vi "RobAndVision Calib.vi"() -> ()   [LabVIEW 2019]
uses:
  VisionSet/System/Ctrl/Photo.ctl
  VisionSet/System/Ctrl/Snap.ctl
  VisionSet/System/Ctrl/Grab.ctl
  <vilib>/vision/Image Controls.llb/IMAQ Image.ctl
  <vilib>/Utility/miscctls.llb/LVPositionTypeDef.ctl
  VisionSet/System/iVision/Controls/Parameter.ctl
  <vilib>/vision/Calibration.llb/Calibration Reference Points.ctl
  <vilib>/vision/Calibration.llb/Distortion Model.ctl
  <vilib>/vision/Calibration.llb/Distortion Model Types.ctl
  82d71f7b-eff0-4029-865a-31d7ef133adf.vi
  f2c65bda-5532-4734-abd4-11d5f743d3e2.vi
  7fbe03bc-4cd6-46c6-99fb-193606e1ede5.vi
  cee5a01b-f54d-48e6-866c-d4c8b1824800.vi
  57e8f32b-8e96-48c7-8808-a32c069fc57f.vi
  0d2cf41f-4f59-416b-aed8-33cf38611db5.vi
  d4251633-b06f-41b2-8266-4a47a039af55.vi
  f1238aa0-85ca-4192-9bd4-185fb6dc1a45.vi
  9afc25ec-97d4-45e3-b1ed-0db5aa0ecab6.vi
  3be21112-cc0e-4c3e-822b-1ce693b2e410.vi
  4e0eac2e-4d25-4abe-97ec-9d7757f58109.vi
  <vilib>/JDP Science/JSONtext/JSON text to Variant.vi
  VisionSet/System/iVision/Global/VisionGlb.vi
  <vilib>/JDP Science/JSONtext/Variant to JSON Text.vi
  LLB/Commonly VI.lvlib
  <vilib>/vision/NI_Vision_Development_Module.lvlib
panel:
  in  "Interpolation Type":u32(ring) items=["Zero Order", "Bi-Linear", "Quadratic", "Cubic Spline"]
  out "Calib Tem":T1
  in  "Seek Forward Button":bool
  in  "Seek Back Button":bool
  in  "Tab Control":enum32{"Page 1", "Page 2"}(tab)
  in  "Tab Control 3":enum32{"檢測圖", "校正圖"}(tab)
  out "Image":T1(plugin-control)
  out "Image 2":T1(plugin-control)
  in  "Btn_Save":bool
  in  "btn_Grab":T2
  in  "Btn_Snap":T3
  in  "Tab Control 2":enum32{"ToolData", "Vision&Robot"}(tab)
  in  "Tab Step":enum32{"Step1"}(tab)
  in  "ToolData":cluster{"X":dbl, "Y":dbl, "Angle":dbl}
  in  "RobotPos 2":cluster{"X":dbl, "Y":dbl, "Angle":dbl}
  in  "RobotPos 1":cluster{"X":dbl, "Y":dbl, "Angle":dbl}
  in  "UseCalib":bool caption="使用手臂坐標輸出"
  in  "ImgCalibration":bool caption="圖像校正"
  in  "PointName":u16(ring) caption="點位名稱" items=["1", "2", "3", "4", "5", "6", "7", "8", "9"]
  in  "btn_Search":bool
  in  "ProjectSet":u16(ring) caption="檢測設定專案"
  in  "Vision&Robot":T4(array[cluster])=[{"VisionPoint"={"X"=1142.846313, "Y"=534.709839}, "RobotPoint"={"X"=148.382, "Y"=73.831, "U"=0.0}}, {"VisionPoint"={"X"=2874.444336, "Y"=544.788269}, "RobotPoint"={"X"=351.458, "Y"=80.442, "U"=0.0}}, {"VisionPoint"={"X"=1132.611328, "Y"=1805.647461}, "RobotPoint"={"X"=152.021, "Y"=-80.98, "U"=0.0}}, {"VisionPoint"={"X"=2866.671875, "Y"=1821.208374}, "RobotPoint"={"X"=356.701, "Y"=-71.332, "U"=0.0}}, {"VisionPoint"={"X"=0.0, "Y"=0.0}, "RobotPoint"={"X"=0.0, "Y"=0.0, "U"=0.0}}, {"VisionPoint"={"X"=0.0, "Y"=0.0}, "RobotPoint"={"X"=0.0, "Y"=0.0, "U"=0.0}}, {"VisionPoint"={"X"=0.0, "Y"=0.0}, "RobotPoint"={"X"=0.0, "Y"=0.0, "U"=0.0}}]
  in  "相機":u16(ring) items=["cam0"]
  in  "Photo":T5
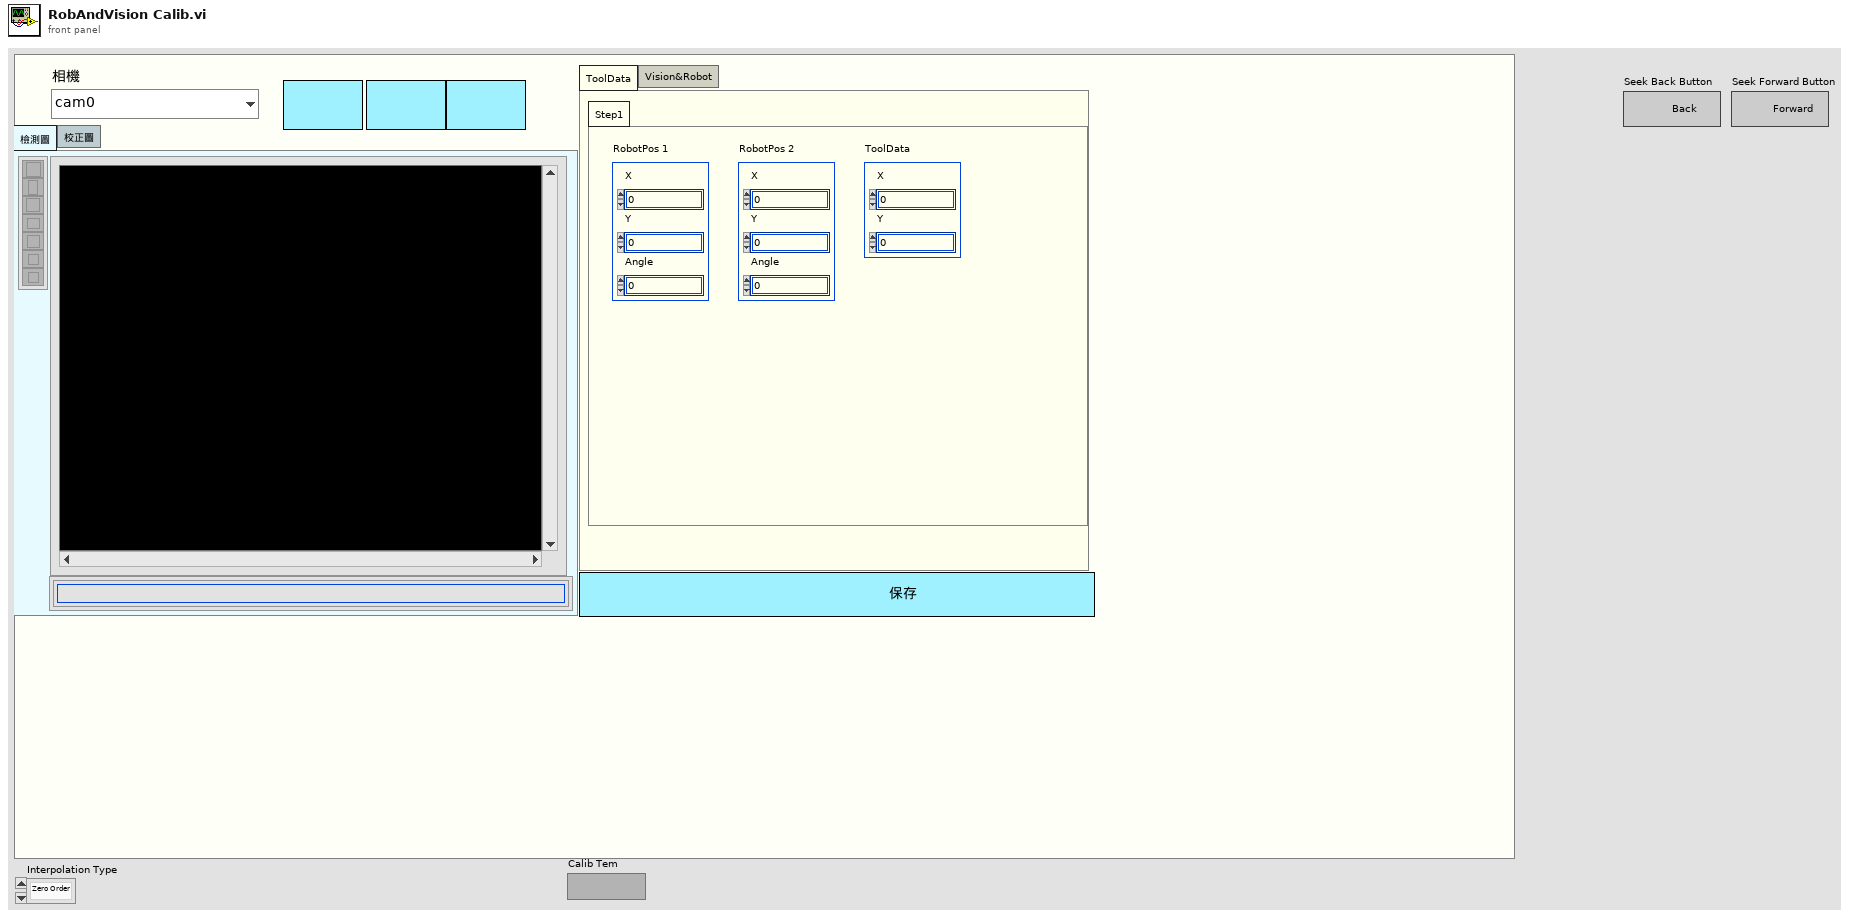
[diagram p1: front panel]
types:
  T1 = typedef "IMAQ Image.ctl" = refnum<image>
  T2 = typedef "Grab.ctl" = bool
  T3 = typedef "Snap.ctl" = bool
  T4 = cluster{"VisionPoint":cluster{"X":dbl, "Y":dbl}, "RobotPoint":cluster{"X":dbl, "Y":dbl, "U":dbl}}[]
  T5 = typedef "Photo.ctl" = bool
  T6 = typedef "LVPositionTypeDef.ctl" = cluster{"Left":i32, "Top":i32}
  T7 = enum16{"Initial", "Write", "Read", "Save", "Load", "WrteAll"}
  T8 = enum16{"initial", "write", "add", "delete", "Load", "Save", "Read", "ReadProjectName"}
  T9 = typedef "Parameter.ctl" = enum16{"Initialize", "Write", "Read", "WriteAll", "Save", "Load"}
  T10 = typedef "Distortion Model.ctl" = cluster{"Distortion Model":T11, "Polynomial Model Setup":cluster{"Radial Coefficient":u32, "Tangential Coefficients ":bool}}
  T11 = typedef "Distortion Model Types.ctl" = i32
  T12 = typedef "Image Unit" = enum32{"Undefined", "Angström", "Micrometer", "Millimeter", "Centimeter", "Meter", "Kilometer", "Microinch", "Inch", "Feet", "Nautical miles", "Standard miles", "Steps"}
  T13 = typedef "Calibration Reference Points.ctl" = cluster{"Pixel Coordinates":cluster{"X":dbl, "Y":dbl}[], "Real World Coordinates":cluster{"X":dbl, "Y":dbl}[], "Unit":T12, "Image Size":cluster{"X":u32, "Y":u32}}
  T14 = typedef "Image Type" = u32
  T15 = cluster{"0 Angle X Tool":dbl, "0 Angle Y Tool":dbl, dbl}
  T16 = typedef "ParameterData.ctl" = cluster{"Rotate Angle":dbl, "Rotate?":bool, "Calibration File Path":string, "Cal?":bool}
  T17 = cluster{"ProjectName":string, "Parameter":string[][]}
  T18 = cluster{"ROI":string, "Numbers":i32, "Data":string[][]}[]
  T19 = cluster{"VisionPoint":cluster{"X":dbl, "Y":dbl}, "RobotPoint":cluster{"X":dbl, "Y":dbl, "U":dbl}}
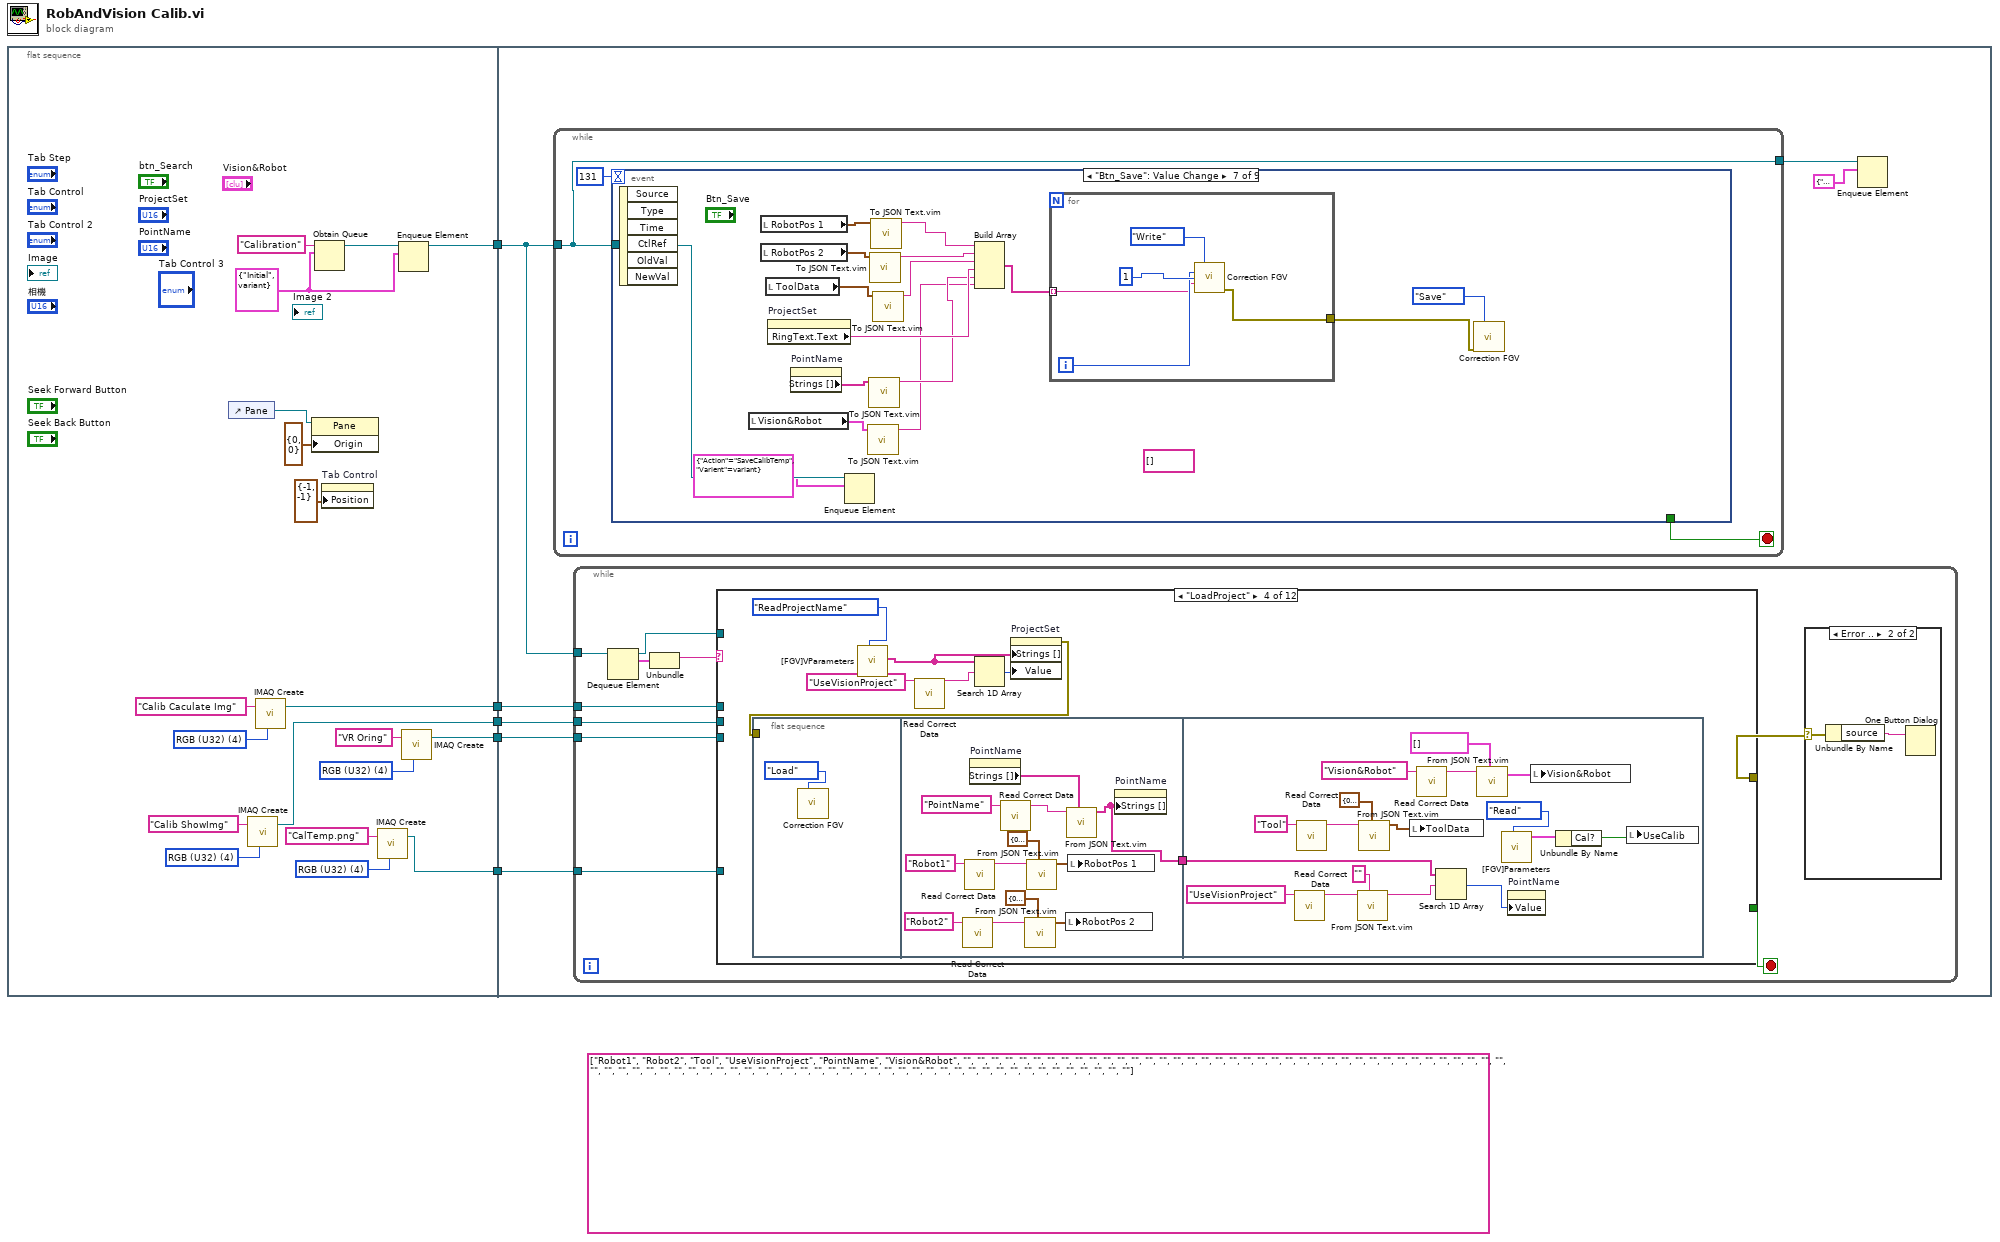
[diagram p0: block diagram]
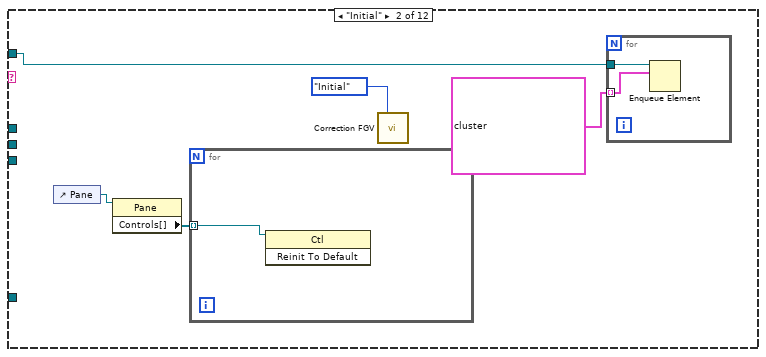
[diagram p4: hidden frame]
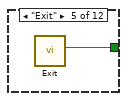
[diagram p6: hidden frame]
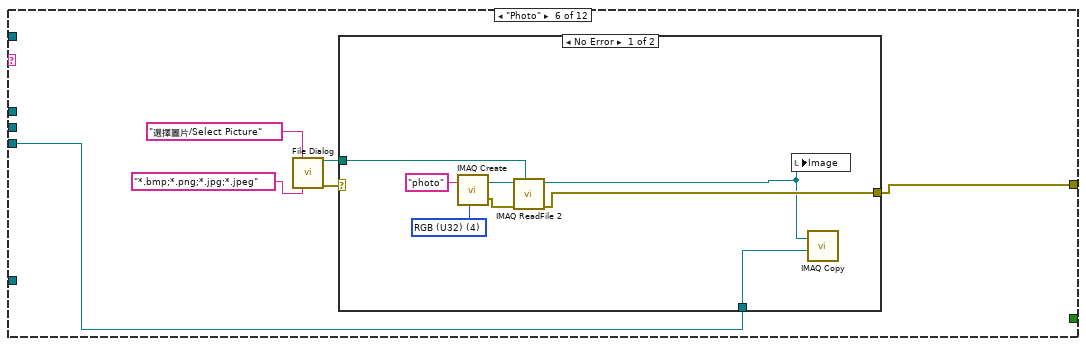
[diagram p7: hidden frame]
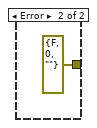
[diagram p8: hidden frame]
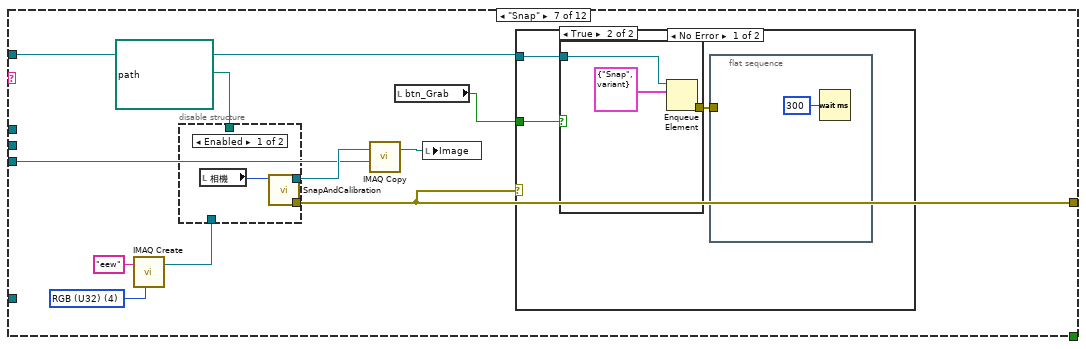
[diagram p9: hidden frame]
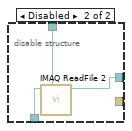
[diagram p10: hidden frame]
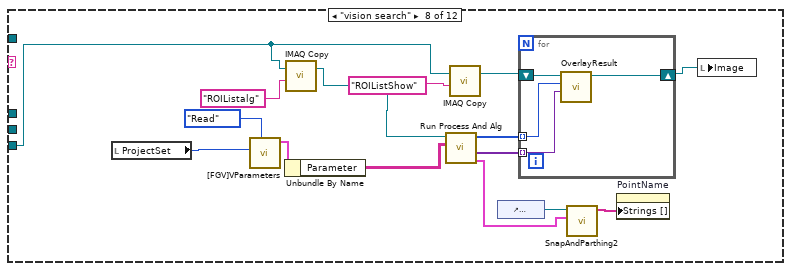
[diagram p13: hidden frame]
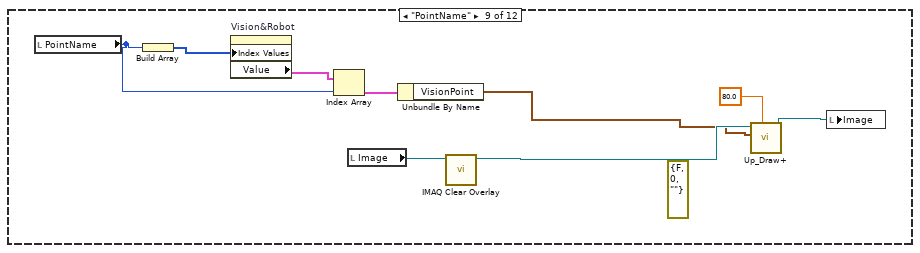
[diagram p14: hidden frame]
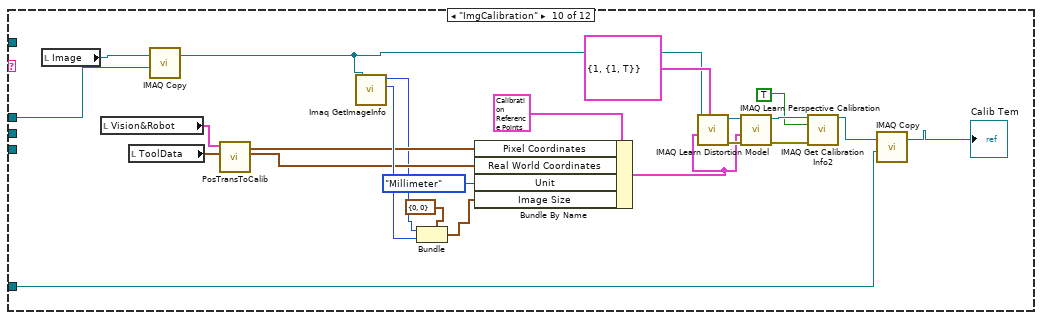
[diagram p15: hidden frame]
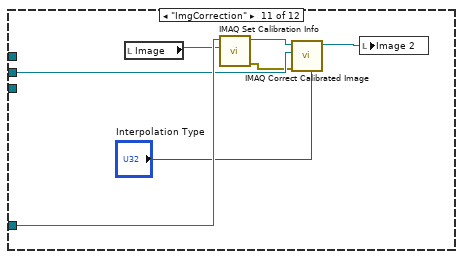
[diagram p16: hidden frame]
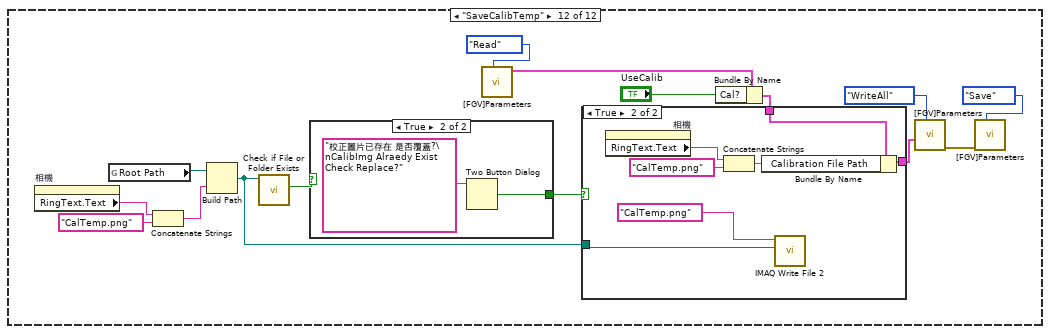
[diagram p17: hidden frame]
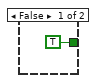
[diagram p19: hidden frame]
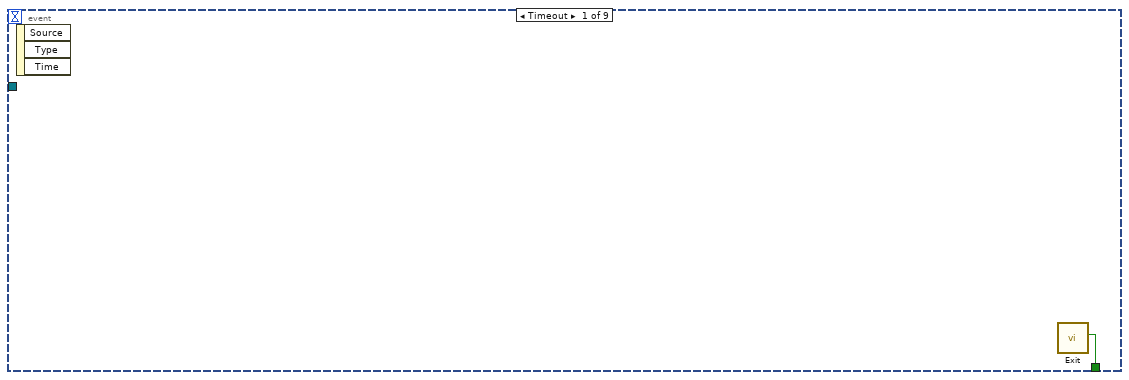
[diagram p20: hidden frame]
diagram:
  (unwired) string[][] [["Robot1", "Robot2", "Tool", "UseVisionProject", "PointName", "Vision&Robot", "", "", "", "", "", "", "", "", "", "", "", "", "", "", ""], ["", "", "", "", "", "", "", "", "", "", "", "", "", "", "", "", "", "", "", "", ""], ["", "", "", "", "", "", "", "", "", "", "", "", "", "", "", "", "", "", "", "", ""], ["", "", "", "", "", "", "", "", "", "", "", "", "", "", "", "", "", "", "", "", ""]] ("Item Names")
  n1 = flat-sequence {
    tunnel: [w22] -> w5
    tunnel: [w18] -> w4
    tunnel: [w12] -> w3
    tunnel: [w9] -> w2
    tunnel: [w6] -> w1
    tunnel: w5 -> [w30]
    tunnel: w4 -> [w28]
    tunnel: w3 -> [w27]
    tunnel: w2 -> [w26]
    tunnel: w1 -> [w25]
    frame #0 {
      w8 = T14 4 items=["Grayscale (U8)", "Grayscale (I16)", "Grayscale (SGL)", "Complex (CSG)", "RGB (U32)", "HSL (U32)", "RGB (U64)", "Grayscale (U16)"] ("Image Type")
      w10 = T14 4 items=["Grayscale (U8)", "Grayscale (I16)", "Grayscale (SGL)", "Complex (CSG)", "RGB (U32)", "HSL (U32)", "RGB (U64)", "Grayscale (U16)"] ("Image Type")
      w14 = T14 4 items=["Grayscale (U8)", "Grayscale (I16)", "Grayscale (SGL)", "Complex (CSG)", "RGB (U32)", "HSL (U32)", "RGB (U64)", "Grayscale (U16)"] ("Image Type")
      w19 = T14 4 items=["Grayscale (U8)", "Grayscale (I16)", "Grayscale (SGL)", "Complex (CSG)", "RGB (U32)", "HSL (U32)", "RGB (U64)", "Grayscale (U16)"] ("Image Type")
      w21 = cluster{"Action":string, "Varient":variant} {"Action"="Initial", "Varient"=variant} ("element")
      n2 = control-ref of="Pane"() -> (w17:refnum<vi>)
      n3 = call "IMAQ Create"("Image Name"="Calib ShowImg", "Image Type"=w8) -> ("New Image"=w6:T1)  [unwired: 3 in, 1 out]
      n4 = call "IMAQ Create"("Image Name"="Calib Caculate Img", "Image Type"=w10) -> ("New Image"=w9:T1)  [unwired: 3 in, 1 out]
      n5 = property class="Pane"(reference=w17, "Origin"=T6 {"Left"=0, "Top"=0} ("Position")) -> ()  [unwired: 1 in, 2 out]
      n6 = Obtain Queue(name (unnamed)="Calibration", element data type=w21) -> (queue out=w23:refnum<queue>)  [unwired: 3 in, 2 out]
      n7 = property on="Tab Control" class="TabCtl (strict)"("Position"=T6 {"Left"=-1, "Top"=-1}) -> ()  [unwired: 2 in, 2 out]
      n8 = call "IMAQ Create"("Image Name"="CalTemp.png", "Image Type"=w14) -> ("New Image"=w12:T1)  [unwired: 3 in, 1 out]
      n9 = Enqueue Element(queue=w23, element=w21) -> (queue out=w22:refnum<queue>)  [unwired: 2 in, 2 out]
      n10 = call "IMAQ Create"("Image Name"="VR Oring", "Image Type"=w19) -> ("New Image"=w18:T1)  [unwired: 3 in, 1 out]
    }
    frame #1 {
      n11 = while {
        tunnel: w30 -> [w212]
        tunnel: [w212] -> w31
        stop <- w214 stop-if-true
        n12 = event shown="[6] \"Btn_Save\": Value Change" {
          selector: _ -> [_ _ _ _ _ _ _ _ _]
          dyn-events: _ -> [_ _ _ _ _ _ _ _ _]
          timeout: 131 -> [_ _ _ _ _ _ _ _ _]
          tunnel: [w215 _ _ _ _ _ _ _ _] -> w214
          tunnel: w212 -> [_ w218 w220 w222 w224 w226 w230 _ w257]
          event Timeout {
            n13 = event-data() -> ()  [unwired: 1 in, 3 out]
            n14 = call "Exit.vi"() -> ("ExitOut"=w215:bool)  [unwired: 11 in]
          }
          event "btn_Search": Value Change {
            n15 = event-data() -> ()  [unwired: 1 in, 2 out]
            n16 = local write "btn_Grab"(T2 FALSE ("btn_Grab")) -> ()
            n17 = Enqueue Element(queue=w218, element=cluster{"Action":string, "Varient":variant} {"Action"="vision search", "Varient"=variant}) -> ()  [unwired: 2 in, 3 out]
          }
          event Value Change {
            n18 = event-data() -> ()  [unwired: 1 in, 6 out]
            n19 = Enqueue Element(queue=w220, element=cluster{"Action":string, "Varient":variant} {"Action"="Snap", "Varient"=variant}) -> ()  [unwired: 2 in, 3 out]
          }
          event Value Change {
            n20 = event-data() -> ()  [unwired: 1 in, 6 out]
            n21 = Enqueue Element(queue=w222, element=cluster{"Action":string, "Varient":variant} {"Action"="Snap", "Varient"=variant}) -> ()  [unwired: 2 in, 3 out]
          }
          event Value Change {
            n22 = event-data() -> ()  [unwired: 1 in, 1 out]
            n23 = Enqueue Element(queue=w224, element=cluster{"Action":string, "Varient":variant} {"Action"="Photo", "Varient"=variant}) -> ()  [unwired: 2 in, 3 out]
          }
          event "PointName": Value Change {
            n24 = event-data() -> ()  [unwired: 1 in, 3 out]
            n25 = Enqueue Element(queue=w226, element=cluster{"Action":string, "Varient":variant} {"Action"="PointName", "Varient"=variant}) -> ()  [unwired: 2 in, 3 out]
          }
          event "Btn_Save": Value Change {
            (unwired) string[] [] ("appended array")
            n26 = event-data() -> ()  [unwired: 1 in, 6 out]
            n27 = local read "Vision&Robot"() -> (w238:T4)
            n28 = local read "RobotPos 1"() -> (w242:cluster{"X":dbl, "Y":dbl, "Angle":dbl})
            n29 = local read "RobotPos 2"() -> (w241:cluster{"X":dbl, "Y":dbl, "Angle":dbl})
            n30 = local read "ToolData"() -> (w240:cluster{"X":dbl, "Y":dbl, "Angle":dbl})
            n31 = property on="ProjectSet" class="Ring (strict)"() -> ("RingText.Text"=w234:string)  [unwired: 2 in, 2 out]
            n32 = property on="PointName" class="Ring (strict)"() -> ("Strings []"=w239:string[])  [unwired: 2 in, 2 out]
            n33 = Enqueue Element(queue=w230, element=cluster{"Action":string, "Varient":variant} {"Action"="SaveCalibTemp", "Varient"=variant}) -> ()  [unwired: 2 in, 3 out]
            n34 = call "To JSON Text.vim"("Anything"=w238) -> ("<JSON>"=w232:string)  [unwired: 9 in, 1 out]
            n35 = call "To JSON Text.vim"("Anything"=w239) -> ("<JSON>"=w233:string)  [unwired: 9 in, 1 out]
            n36 = call "To JSON Text.vim"("Anything"=w241) -> ("<JSON>"=w236:string)  [unwired: 9 in, 1 out]
            n37 = call "To JSON Text.vim"("Anything"=w242) -> ("<JSON>"=w237:string)  [unwired: 9 in, 1 out]
            n38 = call "To JSON Text.vim"("Anything"=w240) -> ("<JSON>"=w235:string)  [unwired: 9 in, 1 out]
            n39 = Build Array(w237, w236, w235, w234, w233, w232) -> (w231:string[])
            n40 = for {
              tunnel: w231 -> [w244] mode=indexing
              tunnel: [w243] -> w227
              i -> [w245]
              n41 = call "Correction FGV.vi"("Action"=T7."Write", "X"=w245, "Y"=1, "DataIn"=w244) -> ("error out"=w243:errorcluster)  [unwired: 9 in, 2 out]
            }
            n42 = call "Correction FGV.vi"("Action"=T7."Save", "error in"=w227) -> ()  [unwired: 11 in, 3 out]
          }
          event "RobotPos 1", "RobotPos 2": Value Change {
            n43 = event-data() -> ()  [unwired: 1 in, 6 out]
            n44 = call "Robot Too Caculate.vi"("RobotPos 2"="RobotPos 2", "RobotPos 1"="RobotPos 1") -> ("0 Angle Y Tool"=w250:dbl, "0 Angle X Tool"=w251:dbl)  [unwired: 8 in]
            n45 = Bundle("0 Angle X Tool"=w251, "0 Angle Y Tool"=w250, 0.0) -> (w249:T15)  [unwired: 1 in]
            n46 = local write "ToolData"(w249) -> ()
          }
          event "ImgCalibration": Value Change {
            n47 = event-data() -> ()  [unwired: 1 in, 2 out]
            n48 = Enqueue Element(queue=w257, element=cluster{"Action":string, "Varient":variant} {"Action"="ImgCalibration", "Varient"=variant}) -> (queue out=w255:refnum<queue>)  [unwired: 2 in, 2 out]
            n49 = Enqueue Element(queue=w255, element=cluster{"Action":string, "Varient":variant} {"Action"="ImgCorrection", "Varient"=variant}) -> ()  [unwired: 2 in, 3 out]
          }
        }
      }
      n50 = while {
        tunnel: w30 -> [w41]
        tunnel: w28 -> [w37]
        tunnel: w27 -> [w34]
        tunnel: w26 -> [w33]
        tunnel: w25 -> [w32]
        stop <- w38 stop-if-true
        n51 = Dequeue Element(queue=w41) -> (queue out=w35:refnum<queue>, element=w40:cluster{"Action":string, "Varient":variant})  [unwired: 2 in, 2 out]
        n52 = Unbundle(w40) -> ("Action"=w39:string)  [unwired: 1 out]
        n53 = case shown="\"LoadProject\"" w39 {
          tunnel: [_ _ _ _ w89 _ _ _ _ _ _ _] -> w38
          tunnel: w37 -> [_ _ _ _ _ w90 w113 w136 _ _ _ _]
          tunnel: [_ _ _ _ _ w91 w111 _ _ _ _ _] -> w36
          tunnel: w35 -> [_ w46 _ _ _ _ w110 _ _ _ _ _]
          tunnel: w34 -> [_ _ _ _ _ _ _ _ _ w163 w185 _]
          tunnel: w33 -> [_ _ _ _ _ _ _ _ _ w160 _ _]
          tunnel: w32 -> [_ _ _ _ _ _ _ _ _ _ w181 _]
          frame "False", Default {
          }
          frame "Initial" {
            n54 = control-ref of="Pane"() -> (w48:refnum<vi>)
            n55 = property class="Pane"(reference=w48) -> ("Controls[]"=w47:refnum<vi>[])  [unwired: 1 in, 2 out]
            n56 = for {
              tunnel: w47 -> [w51] mode=indexing
              n57 = invoke class="Ctl" method="Reinit To Default"(reference=w51) -> ()  [unwired: 2 in, 3 out]
            }
            n58 = call "Correction FGV.vi"("Action"=T7."Initial") -> ()  [unwired: 12 in, 3 out]
            n59 = for {
              tunnel: w46 -> [w50]
              tunnel: cluster{"Action":string, "Varient":variant}[] [{"Action"="GetRoot", "Varient"=variant}, {"Action"="LoadProject", "Varient"=variant}] -> [w49] mode=indexing
              n60 = Enqueue Element(queue=w50, element=w49) -> ()  [unwired: 2 in, 3 out]
            }
          }
          frame "GetRoot" {
          }
          frame "LoadProject" {
            n61 = flat-sequence {
              tunnel: w53 -> [_]
              tunnel: [w60] -> w52
              tunnel: w52 -> [w74]
              frame #0 {
                n62 = call "Correction FGV.vi"("Action"=T7."Load") -> ()  [unwired: 12 in, 3 out]
              }
              frame #1 {
                n63 = call "Read Correct Data.vi"("DataName"="Robot2") -> ("DataOut"=w62:string)  [unwired: 10 in]
                n64 = call "Read Correct Data.vi"("DataName"="Robot1") -> ("DataOut"=w67:string)  [unwired: 10 in]
                n65 = property on="PointName" class="Ring (strict)"() -> ("Strings []"=w69:string[])  [unwired: 2 in, 2 out]
                n66 = call "Read Correct Data.vi"("DataName"="PointName") -> ("DataOut"=w70:string)  [unwired: 10 in]
                n67 = call "From JSON Text.vim"("Data Type and Default Value"=cluster{"X":dbl, "Y":dbl, "Angle":dbl} {"X"=0.0, "Y"=0.0, "Angle"=0.0} ("RobotPos 1"), "JSON"=w62) -> ("Data out"=w64:cluster{"X":dbl, "Y":dbl, "Angle":dbl})  [unwired: 8 in, 1 out]
                n68 = call "From JSON Text.vim"("Data Type and Default Value"=cluster{"X":dbl, "Y":dbl, "Angle":dbl} {"X"=0.0, "Y"=0.0, "Angle"=0.0} ("RobotPos 1"), "JSON"=w67) -> ("Data out"=w65:cluster{"X":dbl, "Y":dbl, "Angle":dbl})  [unwired: 8 in, 1 out]
                n69 = local write "RobotPos 2"(w64) -> ()
                n70 = call "From JSON Text.vim"("Data Type and Default Value"=w69, "JSON"=w70) -> ("Data out"=w60:string[])  [unwired: 8 in, 1 out]
                n71 = local write "RobotPos 1"(w65) -> ()
                n72 = property on="PointName" class="Ring (strict)"("Strings []"=w60) -> ()  [unwired: 2 in, 2 out]
              }
              frame #2 {
                n73 = call "Read Correct Data.vi"("DataName"="UseVisionProject") -> ("DataOut"=w77:string)  [unwired: 10 in]
                n74 = call "Read Correct Data.vi"("DataName"="Tool") -> ("DataOut"=w83:string)  [unwired: 10 in]
                n75 = call "From JSON Text.vim"("Data Type and Default Value"="" ("Ring Text.Text"), "JSON"=w77) -> ("Data out"=w73:string)  [unwired: 8 in, 1 out]
                n76 = call "From JSON Text.vim"("Data Type and Default Value"=cluster{"X":dbl, "Y":dbl, "Angle":dbl} {"X"=0.0, "Y"=0.0, "Angle"=0.0} ("RobotPos 1"), "JSON"=w83) -> ("Data out"=w81:cluster{"X":dbl, "Y":dbl, "Angle":dbl})  [unwired: 8 in, 1 out]
                n77 = local write "ToolData"(w81) -> ()
                n78 = call "Read Correct Data.vi"("DataName"="Vision&Robot") -> ("DataOut"=w87:string)  [unwired: 10 in]
                n79 = Search 1D Array(1D array=w74, element=w73) -> (index of element=w72:i32)  [unwired: 1 in]
                n80 = call "From JSON Text.vim"("Data Type and Default Value"=T4 [] ("Vision&Robot"), "JSON"=w87) -> ("Data out"=w88:T4)  [unwired: 8 in, 1 out]
                n81 = call "[FGV]Parameters.vi"("Parameter"=Parameter."Read") -> ("ParameterData Out"=w79:T16)  [unwired: 9 in, 1 out]
                n82 = property on="PointName" class="Ring (strict)"("Value"=w72) -> ()  [unwired: 2 in, 2 out]
                n83 = local write "Vision&Robot"(w88) -> ()
                n84 = Unbundle By Name(w79) -> ("Cal?"=w78:bool)
                n85 = local write "UseCalib"(w78) -> ()
              }
            }
            n86 = call "[FGV]VParameters.vi"("Enum"=T8."ReadProjectName") -> ("ProjectName"=w54:string[])  [unwired: 7 in, 3 out]
            n87 = call "Read Correct Data.vi"("DataName"="UseVisionProject") -> ("DataOut"=w57:string)  [unwired: 10 in]
            n88 = Search 1D Array(1D array=w54, element=w57) -> (index of element=w56:i32)  [unwired: 1 in]
            n89 = property on="ProjectSet" class="Ring (strict)"("Strings []"=w54, "Value"=w56) -> (error out=w53:errorcluster)  [unwired: 2 in, 1 out]
          }
          frame "Exit" {
            n90 = call "Exit.vi"() -> ("ExitOut"=w89:bool)  [unwired: 11 in]
          }
          frame "Photo" {
            n91 = call "File Dialog"("prompt"="選擇圖片/Select Picture", "pattern (all files)"="*.bmp;*.png;*.jpg;*.jpeg" ("pattern label")) -> ("selected path"=w95:path, "error out"=w94:errorcluster)  [unwired: 10 in, 2 out]
            n92 = case shown="No Error" w94 {
              tunnel: w95 -> [w100 _]
              tunnel: [w98 errorcluster {"status"=FALSE, "code"=0, "source"=""} ("error out")] -> w91
              tunnel: w90 -> [w97 _]
              frame No Error {
                w103 = T14 4 items=["Grayscale (U8)", "Grayscale (I16)", "Grayscale (SGL)", "Complex (CSG)", "RGB (U32)", "HSL (U32)", "RGB (U64)", "Grayscale (U16)"] ("Image Type")
                n93 = call "IMAQ Create"("Image Name"="photo", "Image Type"=w103) -> ("New Image"=w101:T1, "error out"=w99:errorcluster)  [unwired: 3 in]
                n94 = call "IMAQ ReadFile 2"("File Path"=w100, "error in (no error)"=w99, "Image"=w101) -> ("error out"=w98:errorcluster, "Image Out"=w96:T1)  [unwired: 4 in, 3 out]
                n95 = local write "Image"(w96) -> ()
                n96 = call "IMAQ Copy"("Image Dst"=w97, "Image Src"=w96) -> ()  [unwired: 4 in, 2 out]
              }
              frame Error {
              }
            }
          }
          frame "Snap" {
            w107 = T14 4 items=["Grayscale (U8)", "Grayscale (I16)", "Grayscale (SGL)", "Complex (CSG)", "RGB (U32)", "HSL (U32)", "RGB (U64)", "Grayscale (U16)"] ("Image Type")
            n97 = call "IMAQ Create"("Image Name"="eew", "Image Type"=w107) -> ("New Image"=w106:T1)  [unwired: 3 in, 1 out]
            n98 = disable-structure shown="Enabled" {
              disable-tunnel: [w116 w120] -> w114
              disable-tunnel: [w115 _] -> w111
              disable-tunnel: w106 -> [_ w119]
              disable-tunnel: path "C:/Users/USER/Desktop/PATTERN - 複製.png" ("File Path") -> [_ w118]
              frame Enabled {
                n99 = local read "相機"() -> (w117:u16)
                n100 = call "SnapAndCalibration.vi"("Value"=w117) -> ("error out"=w115:errorcluster, "Image Dst Out"=w116:T1)  [unwired: 9 in]
              }
              frame Disabled {
                n101 = call "IMAQ ReadFile 2"("File Path"=w118, "Image"=w119) -> ("Image Out"=w120:T1)  [unwired: 5 in, 4 out]
              }
            }
            n102 = call "IMAQ Copy"("Image Dst"=w113, "Image Src"=w114) -> ("Image Dst Out"=w112:T1)  [unwired: 4 in, 1 out]
            n103 = local read "btn_Grab"() -> (w109:T2)
            n104 = local write "Image"(w112) -> ()
            n105 = case shown="No Error" w111 {
              tunnel: w110 -> [w123 _]
              tunnel: w109 -> [w121 _]
              frame No Error {
                n106 = case shown="True" w121 {
                  tunnel: w123 -> [_ w125]
                  tunnel: [_ w124] -> w122
                  frame False {
                  }
                  frame True {
                    n107 = Enqueue Element(queue=w125, element=cluster{"Action":string, "Varient":variant} {"Action"="Snap", "Varient"=variant}) -> (error out=w124:errorcluster)  [unwired: 2 in, 2 out]
                  }
                }
                n108 = flat-sequence {
                  tunnel: w122 -> [_]
                  frame #0 {
                    n109 = Wait (ms)(milliseconds to wait=u32 300) -> ()  [unwired: 1 out]
                  }
                }
              }
              frame Error {
              }
            }
          }
          frame "vision search" {
            n110 = local read "ProjectSet"() -> (w134:u16)
            n111 = call "[FGV]VParameters.vi"("Enum"=T8."Read", "ProjectIndex"=w134) -> ("DataOut"=w133:T17)  [unwired: 6 in, 3 out]
            n112 = Unbundle By Name(w133) -> ("Parameter"=w132:string[][])
            n113 = call "IMAQ Copy"("Image Dst"="ROIListalg" ("Image Name"), "Image Src"=w136) -> ("Image Dst Out"=w138:T1)  [unwired: 4 in, 1 out]
            n114 = call "Run Process And Alg.vi"("ROIList"=w132, "Image"=w138) -> ("Result Arr"=w129:T18, "DetectOut"=w141:variant[], "AlgOut"=w140:i32[])  [unwired: 5 in, 2 out]
            n115 = call "IMAQ Copy"("Image Dst"="ROIListShow" ("Image Name"), "Image Src"=w136) -> ("Image Dst Out"=w142:T1)  [unwired: 4 in, 1 out]
            n116 = control-ref of="Vision&Robot"() -> (w130:refnum<vi>)
            n117 = for {
              tunnel: w141 -> [w145] mode=indexing
              shift-right: [w144] -> w131
              shift-left: w142 -> [w146]
              tunnel: w140 -> [w143] mode=indexing
              n118 = call "OverlayResult.vi"("DectectResult"=w145, "Algorithm"=w143, "Image"=w146) -> ("Image Out"=w144:T1)  [unwired: 8 in]
            }
            n119 = call "SnapAndParthing2.vi"("Result Arr"=w129, "Vision&Robot"=w130) -> ("Name"=w128:string[])  [unwired: 9 in]
            n120 = property on="PointName" class="Ring (strict)"("Strings []"=w128) -> ()  [unwired: 2 in, 2 out]
            n121 = local write "Image"(w131) -> ()
          }
          frame "PointName" {
            (unwired) errorcluster {"status"=FALSE, "code"=0, "source"=""} ("error out")
            n122 = local read "PointName"() -> (w153:u16)
            n123 = Build Array(w153) -> (w155:u16[])
            n124 = property on="Vision&Robot" class="Arr (strict)"("Index Values"=w155) -> ("Value"=w154:T4)  [unwired: 2 in, 2 out]
            n125 = Index Array(array=w154, index=w153) -> (element=w152:T19)
            n126 = local read "Image"() -> (w151:T1)
            n127 = Unbundle By Name(w152) -> ("VisionPoint"=w149:cluster{"X":dbl, "Y":dbl})
            n128 = call "IMAQ Clear Overlay"("Image"=w151) -> ("Image Out"=w150:T1)  [unwired: 9 in, 1 out]
            n129 = call "Up_Draw+.vi"("y"=80.0, "Center"=w149, "Image"=w150) -> ("Image Out"=w148:T1)  [unwired: 8 in]
            n130 = local write "Image"(w148) -> ()
          }
          frame "ImgCalibration" {
            n131 = local read "Image"() -> (w161:T1)
            n132 = local read "Vision&Robot"() -> (w156:T4)
            n133 = local read "ToolData"() -> (w157:cluster{"X":dbl, "Y":dbl, "Angle":dbl})
            n134 = call "IMAQ Copy"("Image Dst"=w160, "Image Src"=w161) -> ("Image Dst Out"=w159:T1)  [unwired: 4 in, 1 out]
            n135 = call "PosTransToCalib.vi"("ToolData"=w157, "Vision&Robot"=w156) -> ("Real"=w165:cluster{"X":dbl, "Y":dbl}[], "Vision"=w166:cluster{"X":dbl, "Y":dbl}[])  [unwired: 8 in]
            n136 = call "Imaq GetImageInfo"("Image"=w159) -> ("Y Resolution"=w168:i32, "X Resolution"=w158:i32)  [unwired: 3 in, 6 out]
            n137 = Bundle(cluster=cluster{"X":u32, "Y":u32} {"X"=0, "Y"=0} ("Image Size"), "X"=w158, "Y"=w168) -> (w169:cluster{"X":u32, "Y":u32})
            n138 = Bundle By Name(cluster=T13 {"Pixel Coordinates"=[{"X"=1144.0, "Y"=516.0}, {"X"=2876.7, "Y"=527.688}, {"X"=1131.38, "Y"=1786.7}, {"X"=2923.83, "Y"=1804.95}], "Real World Coordinates"=[{"X"=148.386, "Y"=76.831}, {"X"=351.958, "Y"=82.394}, {"X"=152.021, "Y"=-78.481}, {"X"=356.701, "Y"=-69.132}], "Unit"=enum."Millimeter", "Image Size"={"X"=3840, "Y"=2748}} ("Reference Points"), "Pixel Coordinates"=w166, "Real World Coordinates"=w165, "Unit"=Image_Unit."Millimeter", "Image Size"=w169) -> (w171:T13)
            n139 = call "IMAQ Learn Distortion Model"("Distortion Model Setup"=T10 {"Distortion Model"=1, "Polynomial Model Setup"={"Radial Coefficient"=1, "Tangential Coefficients "=TRUE}}, "Reference Points"=w171, "Calibration Template Image"=w159) -> ("error out"=w174:errorcluster, "Calibration Template Image Out"=w177:T1)  [unwired: 3 in, 4 out]
            n140 = call "IMAQ Learn Perspective Calibration"("error in (no error)"=w174, "Reference Points"=w171, "Calibration Template Image"=w177) -> ("error out"=w173:errorcluster, "Calibration Template Image Out"=w176:T1)  [unwired: 1 in, 6 out]
            n141 = call "IMAQ Get Calibration Info2"("Calibration Template Image"=w176, "Return Error Information (False)"=TRUE, "error in (no error)"=w173) -> ("Calibration Template Image (duplicate)"=w164:T1)  [unwired: 12 out]
            n142 = call "IMAQ Copy"("Image Dst"=w163, "Image Src"=w164) -> ("Image Dst Out"=→"Calib Tem":T1)  [unwired: 4 in, 1 out]
          }
          frame "ImgCorrection" {
            n143 = local read "Image"() -> (w184:T1)
            n144 = call "IMAQ Set Calibration Info"("Image Dst"=w184, "Image Src"=w185) -> ("error out"=w179:errorcluster, "Calibrated Image"=w183:T1)  [unwired: 8 in]
            n145 = call "IMAQ Correct Calibrated Image"("Interpolation Type"="Interpolation Type", "error in (no error)"=w179, "Image Dst"=w181, "Image Src"=w183) -> ("Corrected Image"=w182:T1)  [unwired: 6 in, 1 out]
            n146 = local write "Image 2"(w182) -> ()
          }
          frame "SaveCalibTemp" {
            n147 = property on="相機" class="Ring (strict)"() -> ("RingText.Text"=w199:string)  [unwired: 2 in, 2 out]
            n148 = global read "VisionGlb.vi" "Root Path"() -> (w198:path)
            n149 = Concatenate Strings(w199, "CalTemp.png" ("string")) -> (w197:string)
            n150 = Build Path(base path=w198, name or relative path=w197) -> (appended path=w186:path)
            n151 = call <vilib>:"Check if File or Folder Exists.vi"("path"=w186) -> ("file or folder exists?"=w196:bool)  [unwired: 8 in, 2 out]
            n152 = case shown="True" w196 {
              tunnel: [TRUE ("T button?") w210] -> w187
              frame False {
              }
              frame True {
                n153 = Two Button Dialog(message="校正圖片已存在 是否覆蓋?\nCalibImg Alraedy Exist Check Replace?") -> (T button?=w210:bool)  [unwired: 2 in]
              }
            }
            n154 = call "[FGV]Parameters.vi"("Parameter"=Parameter."Read") -> ("ParameterData Out"=w190:T16)  [unwired: 9 in, 1 out]
            n155 = Bundle By Name(cluster=w190, "Cal?"="UseCalib") -> (w189:T16)
            n156 = case shown="True" w187 {
              tunnel: w189 -> [w201 w206]
              tunnel: [w201 w204] -> w188
              tunnel: w186 -> [_ w203]
              frame False {
              }
              frame True {
                n157 = property on="相機" class="Ring (strict)"() -> ("RingText.Text"=w208:string)  [unwired: 2 in, 2 out]
                n158 = Concatenate Strings(w208, "CalTemp.png" ("string")) -> (w205:string)
                n159 = Bundle By Name(cluster=w206, "Calibration File Path"=w205) -> (w204:T16)
                n160 = call-poly "IMAQ Write File 2"("File Path"=w203, "Image"="CalTemp.png" ("Image Name")) -> ()  [unwired: 8 in, 2 out]
              }
            }
            n161 = call "[FGV]Parameters.vi"("Parameter"=Parameter."WriteAll", "ParameterData In"=w188) -> ("Error Out"=w192:errorcluster)  [unwired: 8 in, 1 out]
            n162 = call "[FGV]Parameters.vi"("Parameter"=Parameter."Save", "Error In"=w192) -> ()  [unwired: 8 in, 2 out]
          }
        }
        n163 = case shown="Error .." w36 {
          selector: w36 -> [_ w43]
          frame No Error {
          }
          frame Error {
            n164 = Unbundle By Name(w43) -> ("source"=w42:string)
            n165 = One Button Dialog(message=w42) -> ()  [unwired: 1 in, 1 out]
          }
        }
      }
      n166 = Enqueue Element(queue=w31, element=cluster{"Action":string, "Varient":variant} {"Action"="Exit", "Varient"=variant}) -> ()  [unwired: 2 in, 3 out]
    }
  }
